vi "Preset_Edit_CheckTAGsValid.vi"(9 "Presets-new":T4[](array[typedef]) {"max" format="%#_6p"; "min" format="%#_6p"}, 10 "TAGproperties":T1 {"TAGprop"."TagFunc" format="%08x"; "TAGprop"."RangeL" format="%.2f"; "TAGprop"."RangeH" format="%.2f"}) -> (2 "TAGs OK":bool)   [LabVIEW 2020, in "Sgraph_lib_V1.lvlib" / "Gviewer.lvclass"]
doc: "Check if TAGs are OK according to list of all TAGs"
uses:
  Gviewer.lvclass
  controls/EditTagOneTag.ctl
  DBAL/controls/DBAL_TAGprops.ctl
  DBAL/controls/DBAL_TAGpropEdit.ctl
  Common/controls/typedef_com_TagProp.ctl
  Builds/Sgraph_lib_V1.lvlib
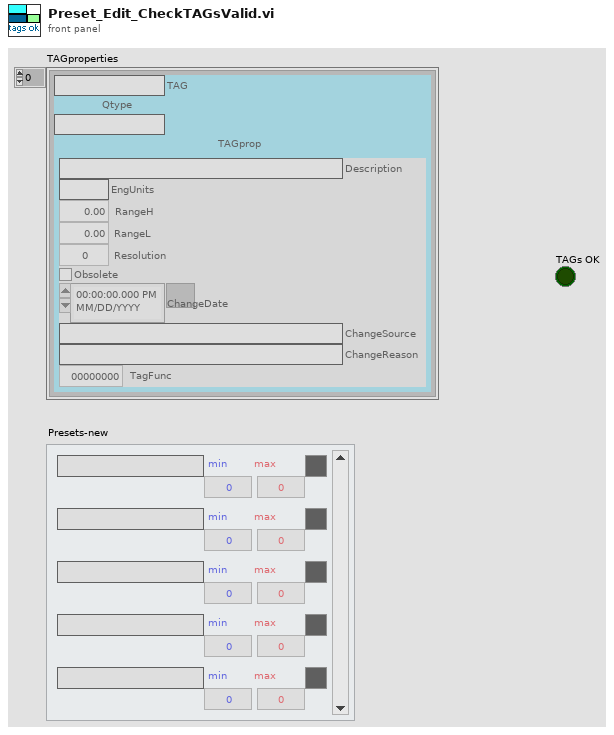
[diagram p1: front panel]
types:
  T1 = typedef "Sgraph_lib_V1.lvlib/DBAL_TAGprops.ctl" = T2[]
  T2 = typedef "Sgraph_lib_V1.lvlib/DBAL_TAGpropEdit.ctl" = cluster{"TAG":string, "Qtype":string, "TAGprop":T3}
  T3 = typedef "Sgraph_lib_V1.lvlib/typedef_com_TagProp.ctl" = cluster{"Description":string, "EngUnits":string, "RangeH":dbl, "RangeL":dbl, "Resolution":i32, "Obsolete":bool, "ChangeDate":timestamp, "ChangeSource":string, "ChangeReason":string, "TagFunc":u32}
  T4 = typedef "Sgraph_lib_V1.lvlib/Gviewer.lvclass/EditTagOneTag.ctl" = cluster{"TAG":string, "min":dbl, "max":dbl, "Color":u32}
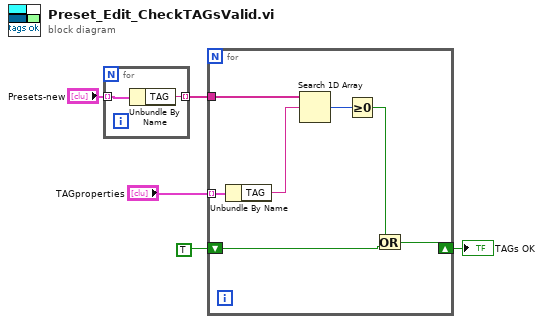
[diagram p0: block diagram]
diagram:
  n1 = for {
    tunnel: "Presets-new" -> [w7] mode=indexing
    tunnel: [w6] -> w3 mode=indexing
    n2 = Unbundle By Name(w7) -> ("TAG"=w6:string)
  }
  n3 = for {
    tunnel: "TAGproperties" -> [w13] mode=indexing
    tunnel: w3 -> [w14]
    shift-right: [w8] -> w1
    shift-left: TRUE -> [w10]
    n4 = Unbundle By Name(w13) -> ("TAG"=w12:string)
    n5 = Search 1D Array(1D array=w14, element=w12) -> (index of element=w11:i32)  [unwired: 1 in]
    n6 = Greater Or Equal To 0?(x=w11) -> (x >= 0?=w9:bool)
    n7 = Or(x=w9, y=w10) -> (x .or. y?=w8:bool)
  }
  "TAGs OK" <- w1
